vi "System4.vi"() -> ()   [LabVIEW 2015]
uses:
  Control 1.ctl
  <vilib>/DAQmx/read.llb/DAQmx Read (Analog 1D Wfm NChan NSamp).vi
  <vilib>/DAQmx/write.llb/DAQmx Write (Digital 1D Bool NChan 1Samp 1Line).vi
  <vilib>/Analysis/baseanly.llb/Mean (DBL).vi
  <vilib>/DAQmx/write.llb/DAQmx Write (Analog DBL 1Chan 1Samp).vi
  <vilib>/DAQmx/miscellaneous.llb/DAQmx Fill In Error Info.vi
  <vilib>/addons/control/pid/NI_PID_autopid.lvlib
  <vilib>/Analysis/NI_AALBase.lvlib
panel:
  in  "Open/Close (Green)":bool
  in  "Open/Close (Blue)":bool
  in  "Stop program":bool
  in  "On/Off":bool
  in  "Manual Control 2":bool
  in  "Voltage setting 2":dbl format="%#_13g"
  out "Voltage Reading(pressure) 2":dbl format="%#_13g"
  out "Pressure 2":dbl format="%#.3g"
  out "Pressure Chart 2":dbl(graph)
  in  "autotuning parameters 2":T1={"controller type"=1, "relay cycles"=3, "relay amplitude"=1.0, "control specification"=2, "PV noise level"=0.1} {"PV noise level" format="%.2f"; "control specification" items=["normal", "fast", "slow"]; "relay amplitude" format="%.2f"; "controller type" items=["PID", "PI", "P"]}
  in  "PID gains 2":T2={"proportional gain (Kc)"=1.0, "integral time (Ti, min)"=0.01, "derivative time (Td, min)"=0.0} {"derivative time (Td, min)" format="%.3f"; "integral time (Ti, min)" format="%.3f"; "proportional gain (Kc)" format="%.3f"}
  out "PID gains out 2":T2={"proportional gain (Kc)"=1.0, "integral time (Ti, min)"=0.01, "derivative time (Td, min)"=0.0} {"derivative time (Td, min)" format="%.3f"; "integral time (Ti, min)" format="%.3f"; "proportional gain (Kc)" format="%.3f"}
  in  "autotune? (F) 2":bool
  in  "reinitialize? (F) 2":bool
  in  "setpoint in Bar 2":dbl format="%#.5f"
  out "Control Value 2":dbl
  in  "Voltage setting":dbl format="%#_13g"
  in  "Manual Control":bool
  out "Control Value":dbl
  in  "setpoint in Bar":dbl format="%#.5f"
  in  "reinitialize? (F)":bool
  in  "autotune? (F)":bool
  out "PID gains out":T2={"proportional gain (Kc)"=1.0, "integral time (Ti, min)"=0.01, "derivative time (Td, min)"=0.0} {"derivative time (Td, min)" format="%.3f"; "integral time (Ti, min)" format="%.3f"; "proportional gain (Kc)" format="%.3f"}
  in  "PID gains":T2={"proportional gain (Kc)"=1.0, "integral time (Ti, min)"=0.01, "derivative time (Td, min)"=0.0} {"derivative time (Td, min)" format="%.3f"; "integral time (Ti, min)" format="%.3f"; "proportional gain (Kc)" format="%.3f"}
  in  "autotuning parameters":T1={"controller type"=1, "relay cycles"=3, "relay amplitude"=1.0, "control specification"=2, "PV noise level"=0.1} {"PV noise level" format="%.2f"; "control specification" items=["normal", "fast", "slow"]; "relay amplitude" format="%.2f"; "controller type" items=["PID", "PI", "P"]}
  out "Pressure Chart":dbl(graph)
  out "Pressure":dbl format="%#.3g"
  out "Voltage Reading(pressure)":dbl format="%#_13g"
  # "Pressure Vessel 2"
  # "Pressure Vessel 1"
  # "Readings"
  # "Controls"
  # "Readings"
  # "Controls"
  # "PID Settings"
  # "51.12139\n\n0.044676"
  # "Valves"
  # "Pump 3"
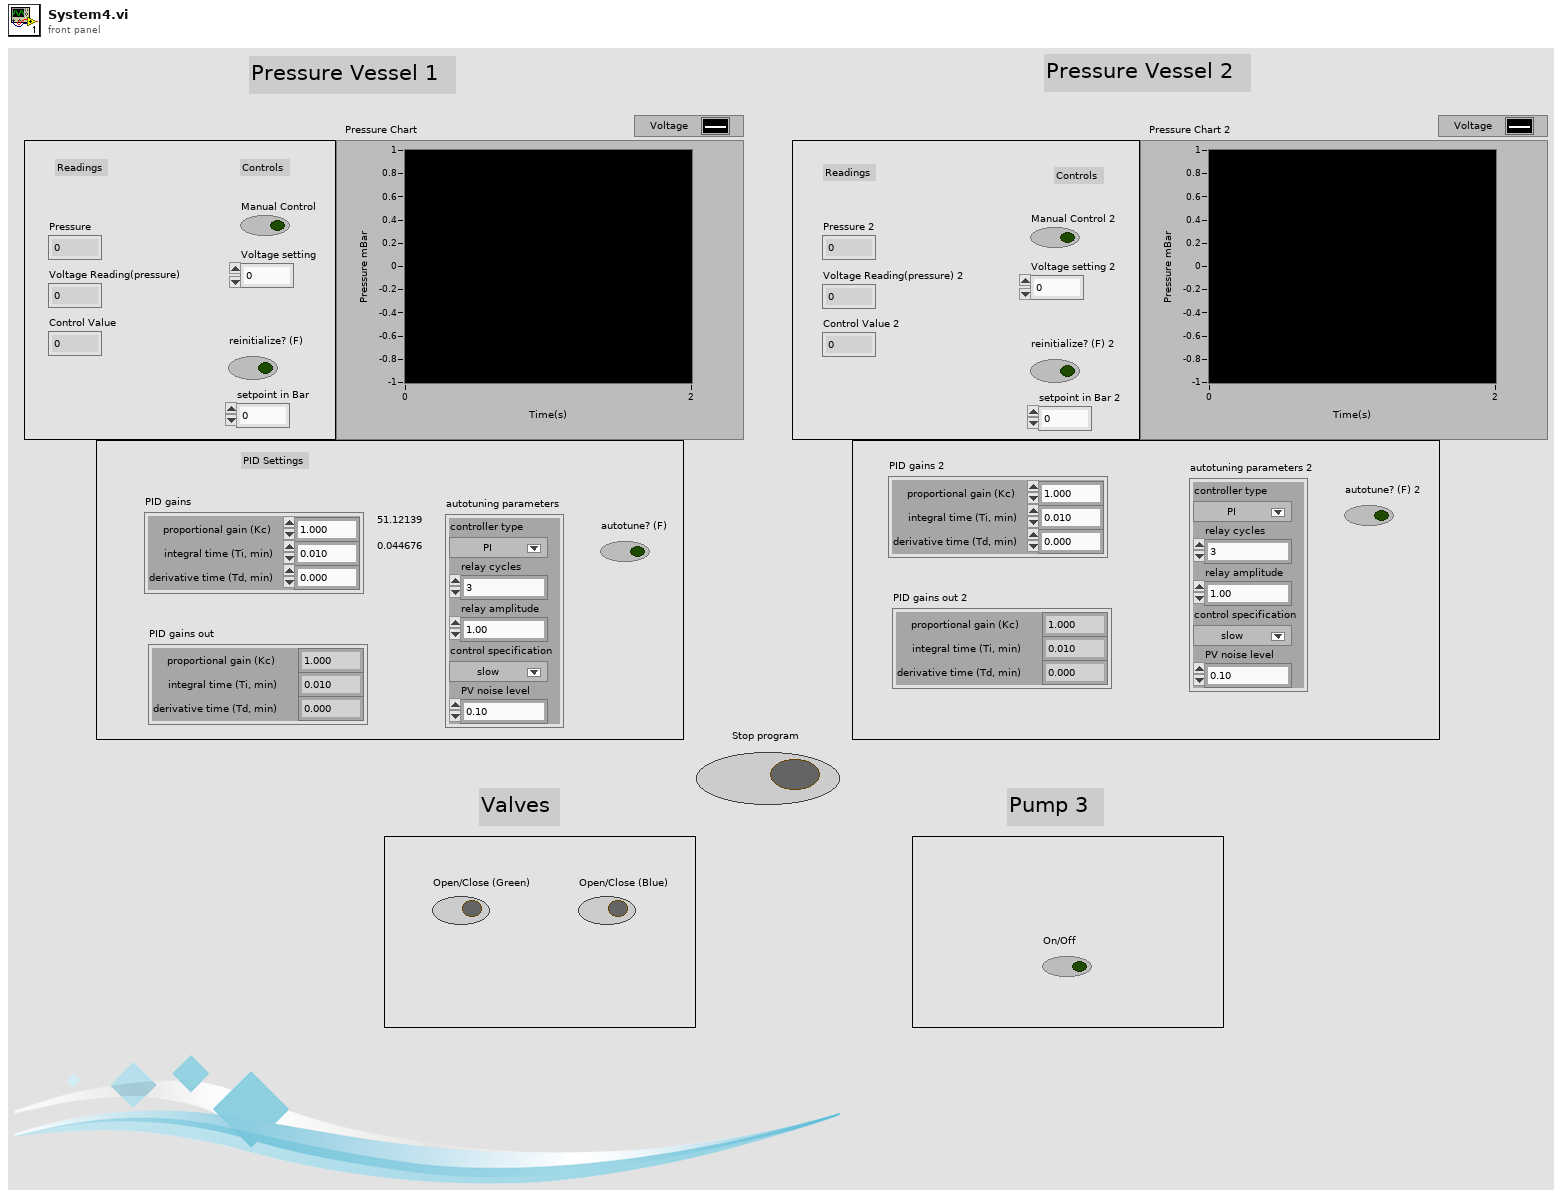
[diagram p1: front panel]
types:
  T1 = cluster{"controller type":u16, "relay cycles":i32, "relay amplitude":dbl, "control specification":u16, "PV noise level":dbl}
  T2 = cluster{"proportional gain (Kc)":dbl, "integral time (Ti, min)":dbl, "derivative time (Td, min)":dbl}
  T3 = typedef "Control 1.ctl" = refnum<k21>
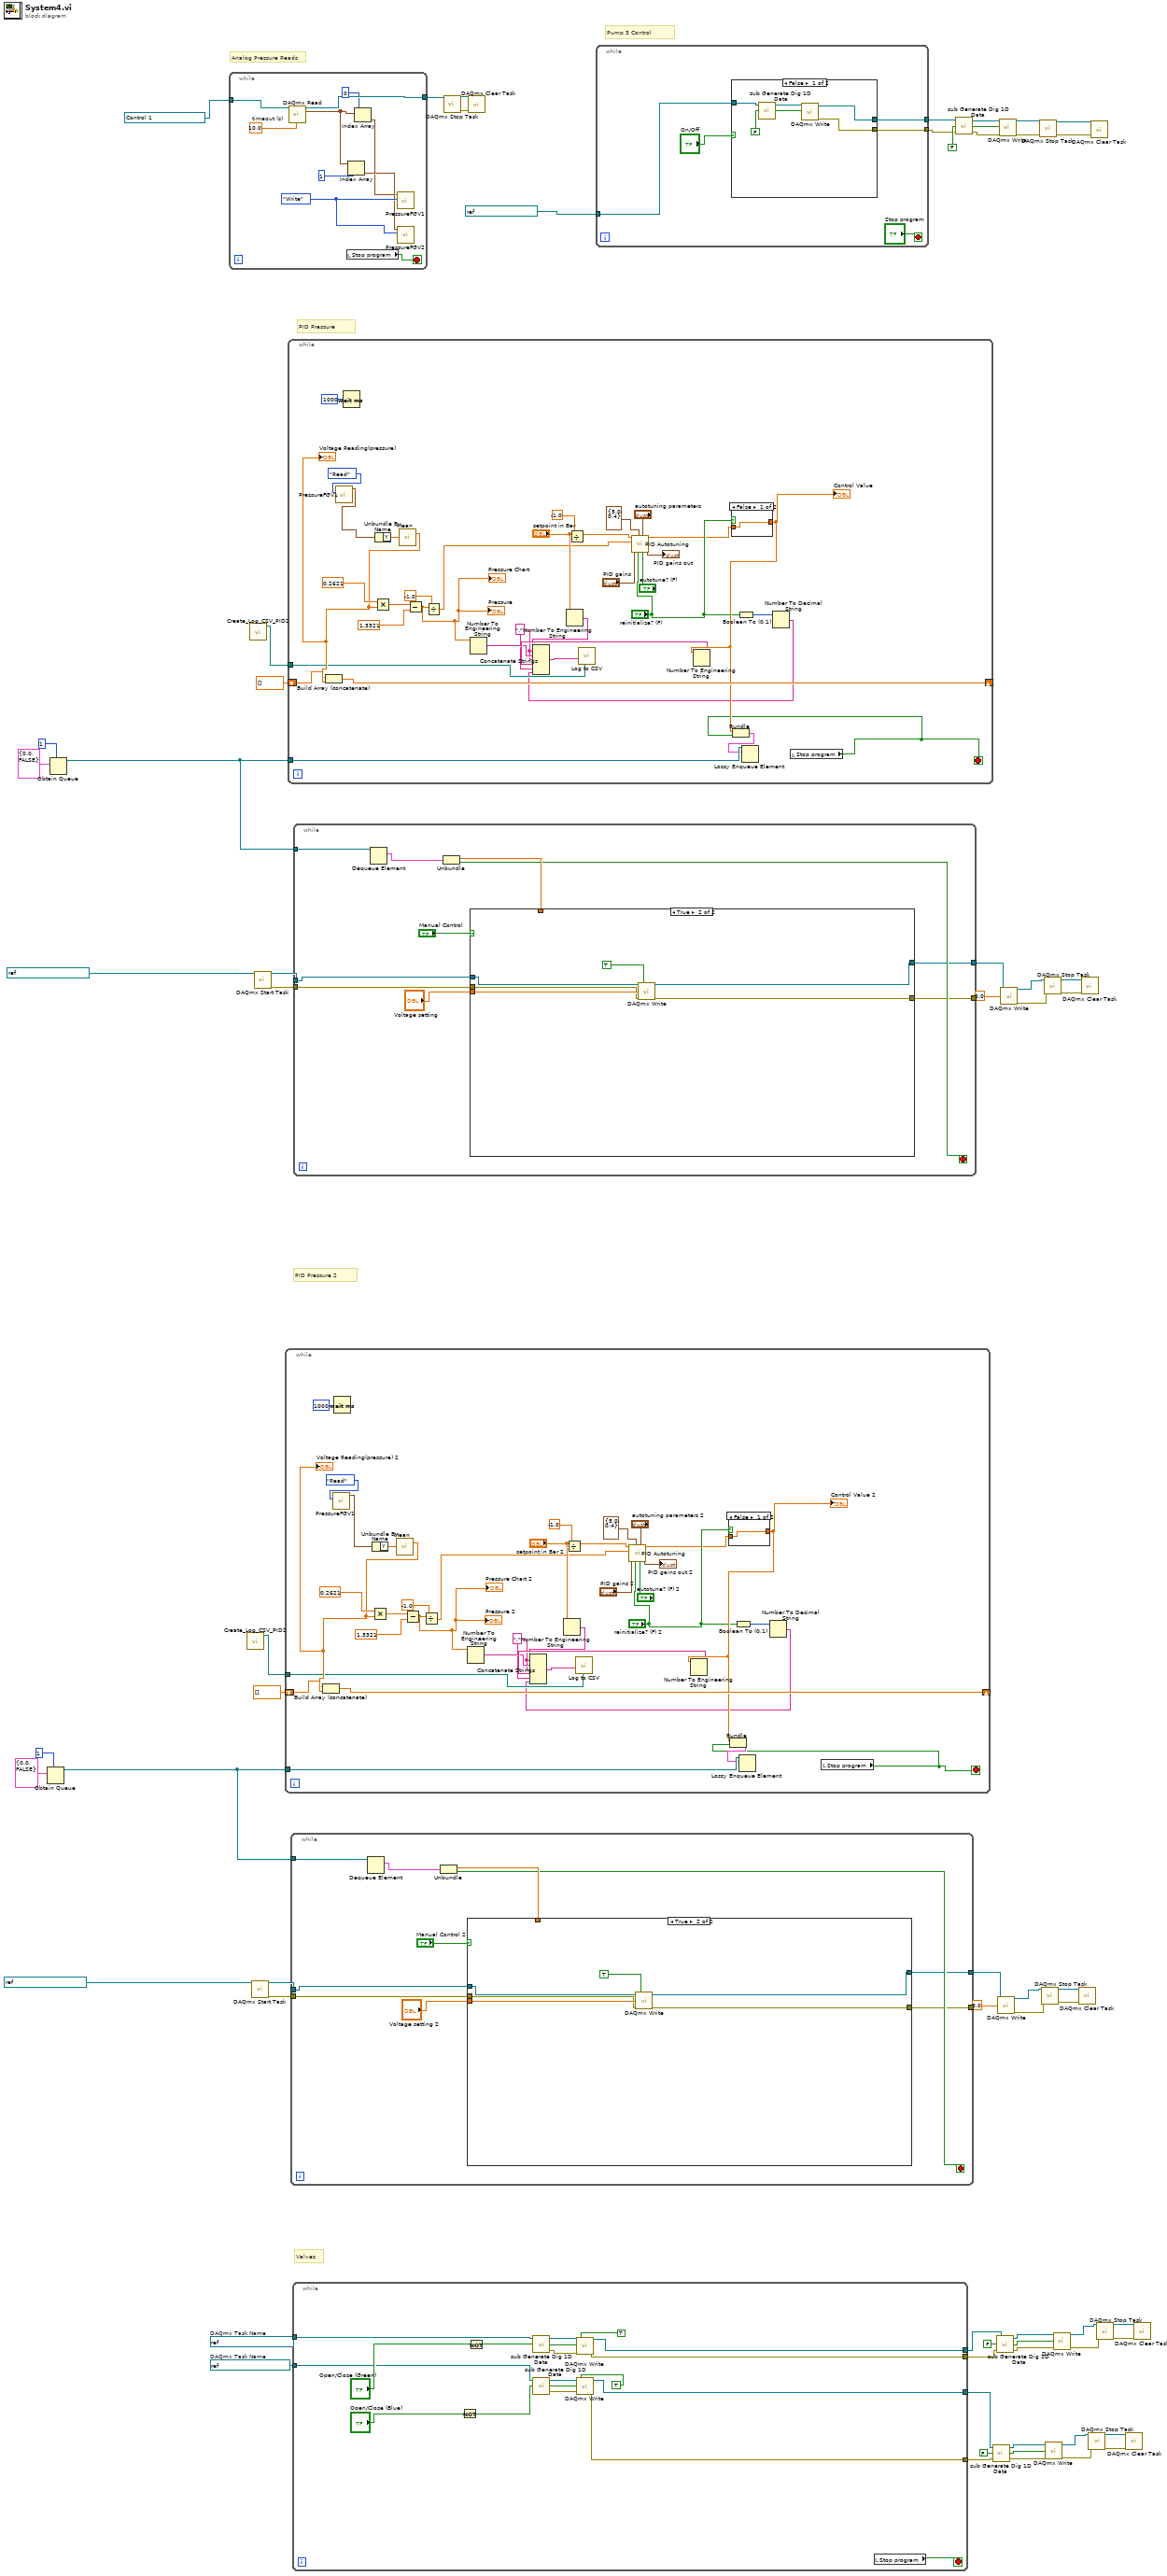
[diagram p0: block diagram]
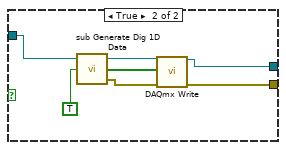
[diagram p2: hidden frame]
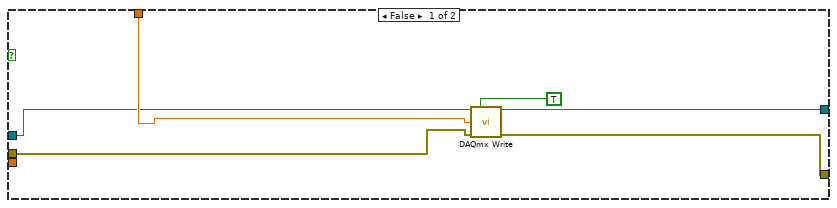
[diagram p3: hidden frame]
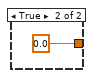
[diagram p4: hidden frame]
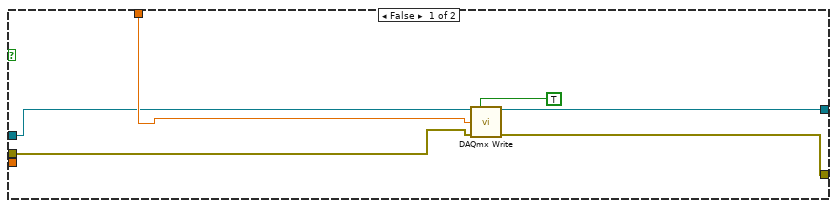
[diagram p5: hidden frame]
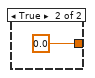
[diagram p6: hidden frame]
diagram:
  w25 = refnum<k21> "NewDigitalSystemBlue"  # DAQmx Task Name
  w26 = refnum<k21> "NewDigitalSystemGreen"  # DAQmx Task Name
  # "Analog Pressure Reads"
  # "Valves"
  # "Pump 3 Control"
  # "PID Pressure"
  # "PID Pressure 2"
  n1 = Obtain Queue(max queue size (-1, unlimited)=1, element data type=cluster{dbl, bool} {0.0, FALSE}) -> (queue out=w50:refnum<queue>)  [unwired: 3 in, 2 out]
  n2 = Obtain Queue(max queue size (-1, unlimited)=1, element data type=cluster{dbl, bool} {0.0, FALSE}) -> (queue out=w64:refnum<queue>)  [unwired: 3 in, 2 out]
  n3 = while {
    tunnel: T3 "New AnalogSystemAI0" -> [w73]
    tunnel: [w72] -> w1
    stop <- w75 stop-if-true
    w68 = enum16{"Write", "Read"}."Write" ("Command")
    w74 = 10.0  # timeout (s)
    n4 = call-poly <vilib>:"DAQmx Read.vi"("task/channels in"=w73, "timeout"=w74) -> ("task out"=w72:refnum<k21>, "data"=w70:waveform(dbl)[])  [unwired: 11 in, 1 out]
    n5 = local read "Stop program"() -> (w75:bool)
    n6 = Index Array(array=w70, index=1) -> (element=w67:waveform(dbl))
    n7 = Index Array(array=w70, index=0) -> (element=w66:waveform(dbl))
    n8 = call "PressureFGV1.vi"("Command"=w68, "element"=w66) -> ()  [unwired: 9 in, 1 out]
    n9 = call "PressureFGV2.vi"("Command"=w68, "element"=w67) -> ()  [unwired: 9 in, 1 out]
  }
  n10 = call "Create_Log_CSV_PID2.vi"() -> ("path"=w46:path)  [unwired: 11 in]
  n11 = call "Create_Log_CSV_PID2.vi"() -> ("path"=w60:path)  [unwired: 11 in]
  n12 = call <vilib>:"DAQmx Start Task.vi"("task/channels in"=refnum<k21> "NewAnalogSystemAO0") -> ("task out"=w45:refnum<k21>, "error out"=w44:errorcluster)  [unwired: 13 in]
  n13 = call <vilib>:"DAQmx Start Task.vi"("task/channels in"=refnum<k21> "NewAnalogSystemAO1") -> ("task out"=w59:refnum<k21>, "error out"=w58:errorcluster)  [unwired: 13 in]
  n14 = while {
    tunnel: w50 -> [w102]
    shift-right: [w99] -> _
    shift-left: dbl[] [] -> [w100]
    tunnel: w46 -> [w93]
    stop <- w80 stop-if-true
    w88 = ","
    n15 = call "PressureFGV1.vi"("Command"=enum16{"Write", "Read"}."Read") -> ("element 2"=w77:waveform(dbl))  [unwired: 10 in]
    n16 = Wait (ms)(milliseconds to wait=u32 1000) -> ()  [unwired: 1 out]
    n17 = Unbundle By Name(w77) -> ("Y"=w76:dbl[])
    n18 = call-poly <vilib>:"Mean.vi"("X"=w76) -> ("mean"=w101:dbl)  [unwired: 1 out]
    "Voltage Reading(pressure) 2" <- w101
    n19 = Build Array (concatenate)(w100, w101) -> (w99:dbl[])
    n20 = Multiply(x=0.2621, y=w101) -> (x*y=w109:dbl)
    n21 = Subtract(x=w109, y=1.3321) -> (x-y=w97:dbl)
    "Pressure 2" <- w97
    "Pressure Chart 2" <- w97
    n22 = Divide(x=w97, y=-1.0) -> (x/y=w85:dbl)
    n23 = Number To Engineering String(4:w97) -> (0:w92:string)  [unwired: 3 in]
    n24 = Number To Engineering String(4:"setpoint in Bar 2") -> (0:w91:string)  [unwired: 3 in]
    n25 = Divide(x="setpoint in Bar 2", y=-1.0) -> (x/y=w84:dbl)
    n26 = call <vilib>:"PID Autotuning.vi"("autotune? (F)"="autotune? (F) 2", "autotuning parameters"="autotuning parameters 2", "reinitialize? (F)"="reinitialize? (F) 2", "output range"=cluster{"output high":dbl, "output low":dbl} {"output high"=5.0, "output low"=0.4}, "PID gains"="PID gains 2", "process variable"=w85, "setpoint"=w84) -> ("PID gains out"=→"PID gains out 2":T2, "output"=w82:dbl)  [unwired: 1 in, 2 out]
    n27 = case shown="False" "reinitialize? (F) 2" {
      tunnel: [w111 0.0] -> w96
      tunnel: w82 -> [w111 _]
      frame False {
      }
      frame True {
      }
    }
    "Control Value 2" <- w96
    n28 = Number To Engineering String(4:w96) -> (0:w95:string)  [unwired: 3 in]
    n29 = Boolean To (0,1)(Boolean="reinitialize? (F) 2") -> (0, 1=w89:i16)
    n30 = Number To Decimal String(number=w89) -> (decimal integer string=w87:string)  [unwired: 1 in]
    n31 = Concatenate Strings(w91, w88, w92, w88, w95, w88, w87) -> (w94:string)
    n32 = call "Log to CSV.vi"("Data Str"=w94, "Path"=w93) -> ()  [unwired: 5 in, 1 out]
    n33 = local read "Stop program"() -> (w80:bool)
    n34 = Bundle("output"=w96, "Stop program"=w80) -> (w81:cluster{"output":dbl, "Stop program":bool})  [unwired: 1 in]
    n35 = Lossy Enqueue Element(queue=w102, element=w81) -> ()  [unwired: 1 in, 4 out]
  }
  n36 = while {
    tunnel: w64 -> [w139]
    shift-right: [w134] -> _
    shift-left: dbl[] [] -> [w135]
    tunnel: w60 -> [w128]
    stop <- w116 stop-if-true
    w123 = ","
    n37 = call "PressureFGV1.vi"("Command"=enum16{"Write", "Read"}."Read") -> ("element 2"=w113:waveform(dbl))  [unwired: 10 in]
    n38 = Wait (ms)(milliseconds to wait=u32 1000) -> ()  [unwired: 1 out]
    n39 = Unbundle By Name(w113) -> ("Y"=w137:dbl[])
    n40 = call-poly <vilib>:"Mean.vi"("X"=w137) -> ("mean"=w136:dbl)  [unwired: 1 out]
    "Voltage Reading(pressure)" <- w136
    n41 = Build Array (concatenate)(w135, w136) -> (w134:dbl[])
    n42 = Multiply(x=0.2621, y=w136) -> (x*y=w146:dbl)
    n43 = Subtract(x=w146, y=1.3321) -> (x-y=w132:dbl)
    "Pressure" <- w132
    "Pressure Chart" <- w132
    n44 = Divide(x=w132, y=-1.0) -> (x/y=w120:dbl)
    n45 = Number To Engineering String(4:w132) -> (0:w127:string)  [unwired: 3 in]
    n46 = Number To Engineering String(4:"setpoint in Bar") -> (0:w126:string)  [unwired: 3 in]
    n47 = Divide(x="setpoint in Bar", y=-1.0) -> (x/y=w119:dbl)
    n48 = call <vilib>:"PID Autotuning.vi"("autotune? (F)"="autotune? (F)", "autotuning parameters"="autotuning parameters", "reinitialize? (F)"="reinitialize? (F)", "output range"=cluster{"output high":dbl, "output low":dbl} {"output high"=5.0, "output low"=0.4}, "PID gains"="PID gains", "process variable"=w120, "setpoint"=w119) -> ("PID gains out"=→"PID gains out":T2, "output"=w117:dbl)  [unwired: 1 in, 2 out]
    n49 = case shown="False" "reinitialize? (F)" {
      tunnel: [w148 0.0] -> w131
      tunnel: w117 -> [w148 _]
      frame False {
      }
      frame True {
      }
    }
    "Control Value" <- w131
    n50 = Number To Engineering String(4:w131) -> (0:w130:string)  [unwired: 3 in]
    n51 = Boolean To (0,1)(Boolean="reinitialize? (F)") -> (0, 1=w124:i16)
    n52 = Number To Decimal String(number=w124) -> (decimal integer string=w122:string)  [unwired: 1 in]
    n53 = Concatenate Strings(w126, w123, w127, w123, w130, w123, w122) -> (w129:string)
    n54 = call "Log to CSV.vi"("Data Str"=w129, "Path"=w128) -> ()  [unwired: 5 in, 1 out]
    n55 = local read "Stop program"() -> (w116:bool)
    n56 = Bundle("output"=w131, "Stop program"=w116) -> (w138:cluster{"output":dbl, "Stop program":bool})  [unwired: 1 in]
    n57 = Lossy Enqueue Element(queue=w139, element=w138) -> ()  [unwired: 1 in, 4 out]
  }
  n58 = while {
    tunnel: w50 -> [w159]
    tunnel: w45 -> [w157]
    tunnel: [w152] -> w42
    tunnel: w44 -> [w151]
    tunnel: [w150] -> _
    stop <- w153 stop-if-true
    n59 = Dequeue Element(queue=w159) -> (element=w156:cluster{dbl, bool})  [unwired: 2 in, 3 out]
    n60 = Unbundle(w156) -> (w155:dbl, w153:bool)
    n61 = case shown="True" "Manual Control 2" {
      tunnel: w157 -> [w163 w170]
      tunnel: w155 -> [w164 _]
      tunnel: "Voltage setting 2" -> [_ w169]
      tunnel: [w162 w168] -> w152
      tunnel: w151 -> [w161 w167]
      tunnel: [w160 w166] -> w150
      frame False {
        n62 = call-poly <vilib>:"DAQmx Write.vi"("task/channels in"=w163, "auto start"=TRUE, "data"=w164, "error in"=w161) -> ("task out"=w162:refnum<k21>, "error out"=w160:errorcluster)  [unwired: 9 in, 1 out]
      }
      frame True {
        n63 = call-poly <vilib>:"DAQmx Write.vi"("task/channels in"=w170, "auto start"=TRUE, "data"=w169, "error in"=w167) -> ("task out"=w168:refnum<k21>, "error out"=w166:errorcluster)  [unwired: 9 in, 1 out]
      }
    }
  }
  n64 = while {
    tunnel: w26 -> [w180]
    tunnel: w25 -> [w179]
    tunnel: [w178] -> w15
    tunnel: [w177] -> w11
    tunnel: [w174] -> w8
    tunnel: [w173] -> w6
    stop <- w172 stop-if-true
    n65 = Not(x="Open/Close (Blue)") -> (.not. x?=w190:bool)
    n66 = Not(x="Open/Close (Green)") -> (.not. x?=w189:bool)
    n67 = call <vilib>:"sub Generate Dig 1D Data.vi"("initial value"=w189, "task in"=w180) -> ("error out"=w176:errorcluster, "Data"=w187:bool[], "task out"=w184:refnum<k21>)  [unwired: 1 in]
    n68 = call <vilib>:"sub Generate Dig 1D Data.vi"("initial value"=w190, "task in"=w179) -> ("error out"=w175:errorcluster, "Data"=w186:bool[], "task out"=w185:refnum<k21>)  [unwired: 1 in]
    n69 = call-poly <vilib>:"DAQmx Write.vi"("task/channels in"=w184, "auto start"=TRUE, "data"=w187, "error in"=w176) -> ("task out"=w178:refnum<k21>, "error out"=w174:errorcluster)  [unwired: 9 in, 1 out]
    n70 = call-poly <vilib>:"DAQmx Write.vi"("task/channels in"=w185, "auto start"=TRUE, "data"=w186, "error in"=w175) -> ("task out"=w177:refnum<k21>, "error out"=w173:errorcluster)  [unwired: 9 in, 1 out]
    n71 = local read "Stop program"() -> (w172:bool)
  }
  n72 = while {
    tunnel: w64 -> [w200]
    tunnel: w59 -> [w198]
    tunnel: [w193] -> w56
    tunnel: w58 -> [w192]
    tunnel: [w191] -> _
    stop <- w194 stop-if-true
    n73 = Dequeue Element(queue=w200) -> (element=w197:cluster{dbl, bool})  [unwired: 2 in, 3 out]
    n74 = Unbundle(w197) -> (w196:dbl, w194:bool)
    n75 = case shown="True" "Manual Control" {
      tunnel: w198 -> [w204 w211]
      tunnel: w196 -> [w205 _]
      tunnel: "Voltage setting" -> [_ w210]
      tunnel: [w203 w209] -> w193
      tunnel: w192 -> [w202 w208]
      tunnel: [w201 w207] -> w191
      frame False {
        n76 = call-poly <vilib>:"DAQmx Write.vi"("task/channels in"=w204, "auto start"=TRUE, "data"=w205, "error in"=w202) -> ("task out"=w203:refnum<k21>, "error out"=w201:errorcluster)  [unwired: 9 in, 1 out]
      }
      frame True {
        n77 = call-poly <vilib>:"DAQmx Write.vi"("task/channels in"=w211, "auto start"=TRUE, "data"=w210, "error in"=w208) -> ("task out"=w209:refnum<k21>, "error out"=w207:errorcluster)  [unwired: 9 in, 1 out]
      }
    }
  }
  n78 = call <vilib>:"DAQmx Stop Task.vi"("task/channels in"=w1) -> ("task out"=w3:refnum<k21>, "error out"=w2:errorcluster)  [unwired: 13 in]
  n79 = call <vilib>:"DAQmx Clear Task.vi"("task in"=w3, "error in"=w2) -> ()  [unwired: 13 in, 1 out]
  n80 = while {
    tunnel: refnum<k21> "NewDigSystemP0L2" -> [w216]
    tunnel: [w215] -> w30
    tunnel: [w214] -> w29
    stop <- "Stop program" stop-if-true
    n81 = case shown="False" "On/Off" {
      tunnel: w216 -> [w223 w227]
      tunnel: [w219 w226] -> w215
      tunnel: [w218 w224] -> w214
      frame False {
        n82 = call <vilib>:"sub Generate Dig 1D Data.vi"("initial value"=FALSE, "task in"=w223) -> ("Data"=w221:bool[], "task out"=w222:refnum<k21>)  [unwired: 1 in, 1 out]
        n83 = call-poly <vilib>:"DAQmx Write.vi"("task/channels in"=w222, "data"=w221) -> ("task out"=w219:refnum<k21>, "error out"=w218:errorcluster)  [unwired: 11 in, 1 out]
      }
      frame True {
        n84 = call <vilib>:"sub Generate Dig 1D Data.vi"("initial value"=TRUE, "task in"=w227) -> ("error out"=w225:errorcluster, "Data"=w229:bool[], "task out"=w228:refnum<k21>)  [unwired: 1 in]
        n85 = call-poly <vilib>:"DAQmx Write.vi"("task/channels in"=w228, "data"=w229, "error in"=w225) -> ("task out"=w226:refnum<k21>, "error out"=w224:errorcluster)  [unwired: 10 in, 1 out]
      }
    }
  }
  n86 = call <vilib>:"sub Generate Dig 1D Data.vi"("error in"=w29, "initial value"=FALSE, "task in"=w30) -> ("error out"=w34:errorcluster, "Data"=w32:bool[], "task out"=w33:refnum<k21>)
  n87 = call <vilib>:"sub Generate Dig 1D Data.vi"("error in"=w6, "initial value"=FALSE, "task in"=w11) -> ("error out"=w5:errorcluster, "Data"=w10:bool[], "task out"=w12:refnum<k21>)
  n88 = call <vilib>:"sub Generate Dig 1D Data.vi"("error in"=w8, "initial value"=FALSE, "task in"=w15) -> ("error out"=w7:errorcluster, "Data"=w9:bool[], "task out"=w16:refnum<k21>)
  n89 = call-poly <vilib>:"DAQmx Write.vi"("task/channels in"=w42, "data"=0.0) -> ("task out"=w41:refnum<k21>, "error out"=w40:errorcluster)  [unwired: 11 in, 1 out]
  n90 = call-poly <vilib>:"DAQmx Write.vi"("task/channels in"=w33, "data"=w32, "error in"=w34) -> ("task out"=w28:refnum<k21>, "error out"=w27:errorcluster)  [unwired: 10 in, 1 out]
  n91 = call-poly <vilib>:"DAQmx Write.vi"("task/channels in"=w56, "data"=0.0) -> ("task out"=w55:refnum<k21>, "error out"=w54:errorcluster)  [unwired: 11 in, 1 out]
  n92 = call <vilib>:"DAQmx Stop Task.vi"("task/channels in"=w28, "error in"=w27) -> ("task out"=w36:refnum<k21>, "error out"=w35:errorcluster)  [unwired: 12 in]
  n93 = call <vilib>:"DAQmx Stop Task.vi"("task/channels in"=w41, "error in"=w40) -> ("task out"=w43:refnum<k21>, "error out"=w39:errorcluster)  [unwired: 12 in]
  n94 = call <vilib>:"DAQmx Stop Task.vi"("task/channels in"=w55, "error in"=w54) -> ("task out"=w57:refnum<k21>, "error out"=w53:errorcluster)  [unwired: 12 in]
  n95 = call-poly <vilib>:"DAQmx Write.vi"("task/channels in"=w12, "data"=w10, "error in"=w5) -> ("task out"=w19:refnum<k21>, "error out"=w18:errorcluster)  [unwired: 10 in, 1 out]
  n96 = call-poly <vilib>:"DAQmx Write.vi"("task/channels in"=w16, "data"=w9, "error in"=w7) -> ("task out"=w22:refnum<k21>, "error out"=w23:errorcluster)  [unwired: 10 in, 1 out]
  n97 = call <vilib>:"DAQmx Clear Task.vi"("task in"=w43, "error in"=w39) -> ()  [unwired: 13 in, 1 out]
  n98 = call <vilib>:"DAQmx Clear Task.vi"("task in"=w57, "error in"=w53) -> ()  [unwired: 13 in, 1 out]
  n99 = call <vilib>:"DAQmx Stop Task.vi"("task/channels in"=w19, "error in"=w18) -> ("task out"=w20:refnum<k21>, "error out"=w17:errorcluster)  [unwired: 12 in]
  n100 = call <vilib>:"DAQmx Clear Task.vi"("task in"=w36, "error in"=w35) -> ()  [unwired: 13 in, 1 out]
  n101 = call <vilib>:"DAQmx Stop Task.vi"("task/channels in"=w22, "error in"=w23) -> ("task out"=w21:refnum<k21>, "error out"=w24:errorcluster)  [unwired: 12 in]
  n102 = call <vilib>:"DAQmx Clear Task.vi"("task in"=w20, "error in"=w17) -> ()  [unwired: 13 in, 1 out]
  n103 = call <vilib>:"DAQmx Clear Task.vi"("task in"=w21, "error in"=w24) -> ()  [unwired: 13 in, 1 out]
